vi "VOC_Multi-Sensor_Data_Logger.vi"() -> ()   [LabVIEW 2021]
uses:
  Program Files (x86)/National Instruments/LabVIEW 2021/examples/Instrument IO/Serial/support/Serial - XON-XOFF Characters.ctl
  Program Files (x86)/National Instruments/LabVIEW 2021/examples/Instrument IO/Serial/support/Serial - ASCII Characters.ctl
  Program Files (x86)/National Instruments/LabVIEW 2021/examples/Instrument IO/Serial/support/Serial - Settings.ctl
  <vilib>/Instr/_visa.llb/VISA Configure Serial Port (Instr).vi
  <vilib>/Utility/file.llb/Write Delimited Spreadsheet (string).vi
  <vilib>/Utility/file.llb/Write Delimited Spreadsheet (DBL).vi
panel:
  out "Elapsed Time (s)":i32
  in  "Log File":path=path "C:/Users/dfdye/Documents/GitHub/VOC_sensor_testing/Data_Logs/Test.tbd"
  in  "Data Logging Interval (sec)":i32=5 min=1 max=3600 step=1
  out "SGP30 TVOC (ppb)":dbl
  out "Humidity (%)":dbl
  out "Pressure (hPa)":dbl
  out "Temperature (deg C)":dbl
  in  "stop":bool
  in  "Serial Port":refnum<visa-resource-name>="COM3"
  out "XY Graph":cluster{i32[], dbl[]}[](graph)
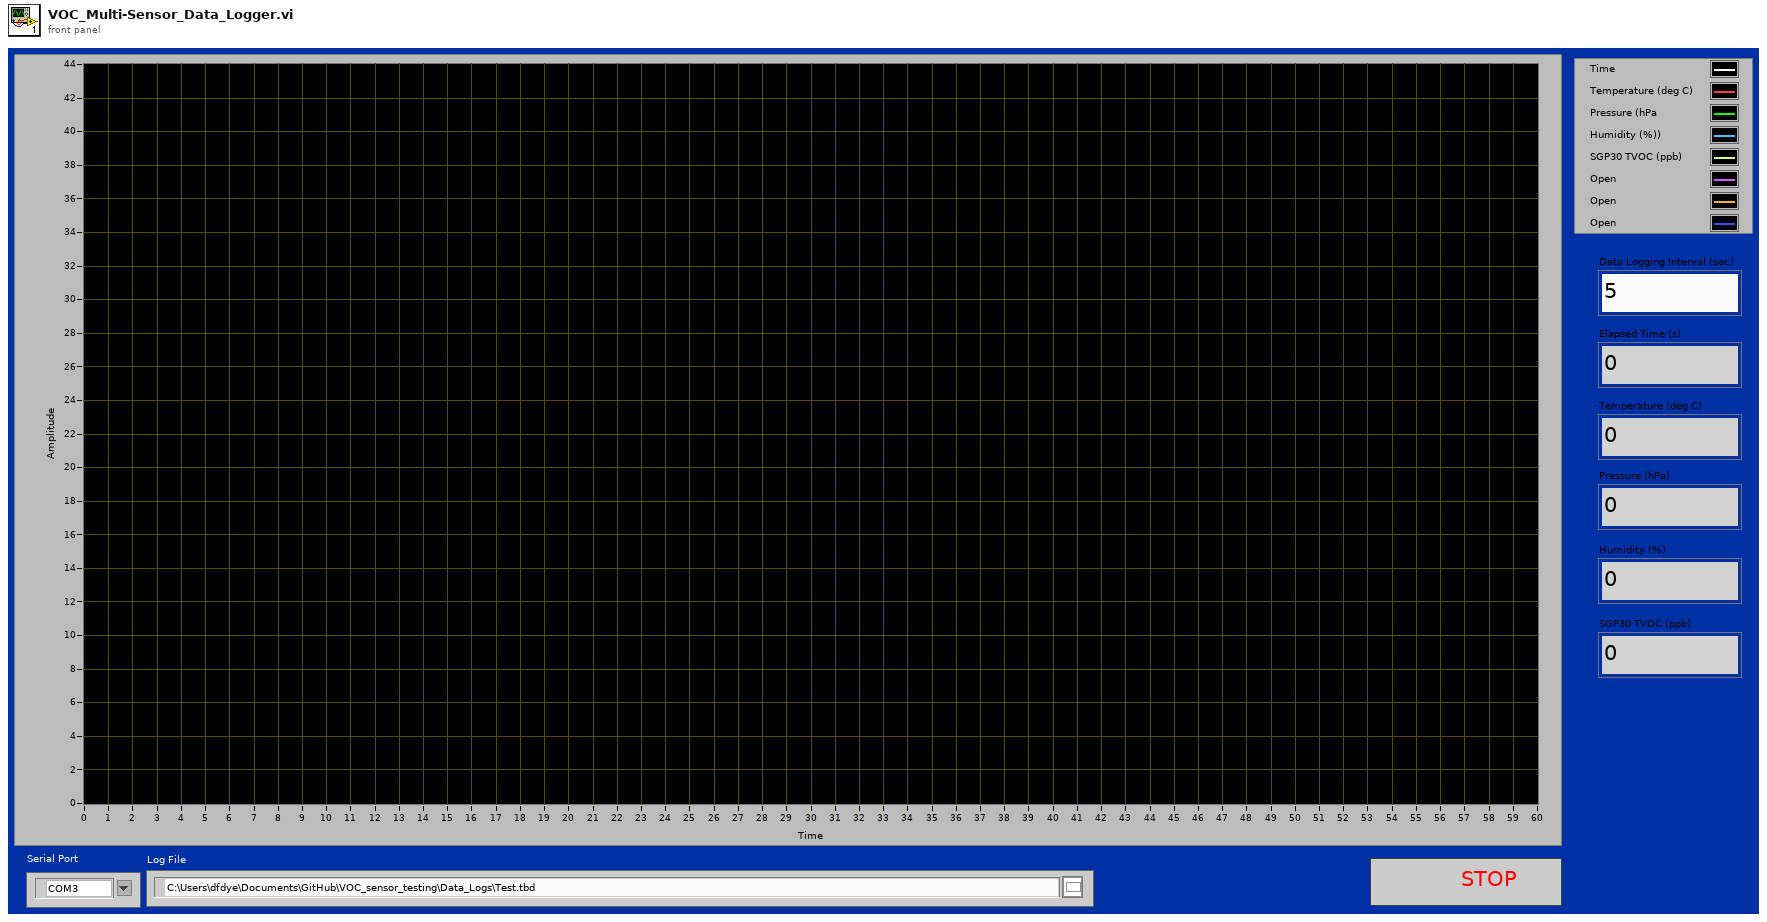
[diagram p1: front panel]
types:
  T1 = typedef "Serial - Settings.ctl" = cluster{"baud rate":u32, "data bits":u16, "parity":enum16{"None", "Odd", "Even", "Mark", "Space"}, "stop bits":u16, "flow control":u16}
  T2 = typedef "Serial - XON-XOFF Characters.ctl" = cluster{"XON":T3, "XOFF":T3}
  T3 = typedef "Serial - ASCII Characters.ctl" = enum16{"NUL", "SOH", "STX", "ETX", "EOT", "ENQ", "ACK", "BEL", "BS", "HT", "LF", "VT", "FF", "CR", "SO", "SI", "DLE", "DC1", "DC2", "DC3", "DC4", "NAK", "SYN", "ETB", "CAN", "EM", "SUB", "ESC", "FS", "GS", "RS", "US", "SP", "!", "\"", "#", "$", "%", "&", "'", "(", ")", "*", "+", ",", "- (-)", ".", "/", "0", "1", "2", "3", "4", "5", "6", "7", "8", "9", ":", ";", "<", "=", ">", "?", "@", "A", "B", "C", "D", "E", "F", "G", "H", "I", "J", "K", "L", "M", "N", "O", "P", "Q", "R", "S", "T", "U", "V", "W", "X", "Y", "Z", "[", "\\", "]", "^", "_", "`", "a", "b", "c", "d", "e", "f", "g", "h", "i", "j", "k", "l", "m", "n", "o", "p", "q", "r", "s", "t", "u", "v", "w", "x", "y", "z", "{", "|", "}", "~"}
  T4 = enum8{"Enabled", "Disabled", "Disabled and Grayed Out"}
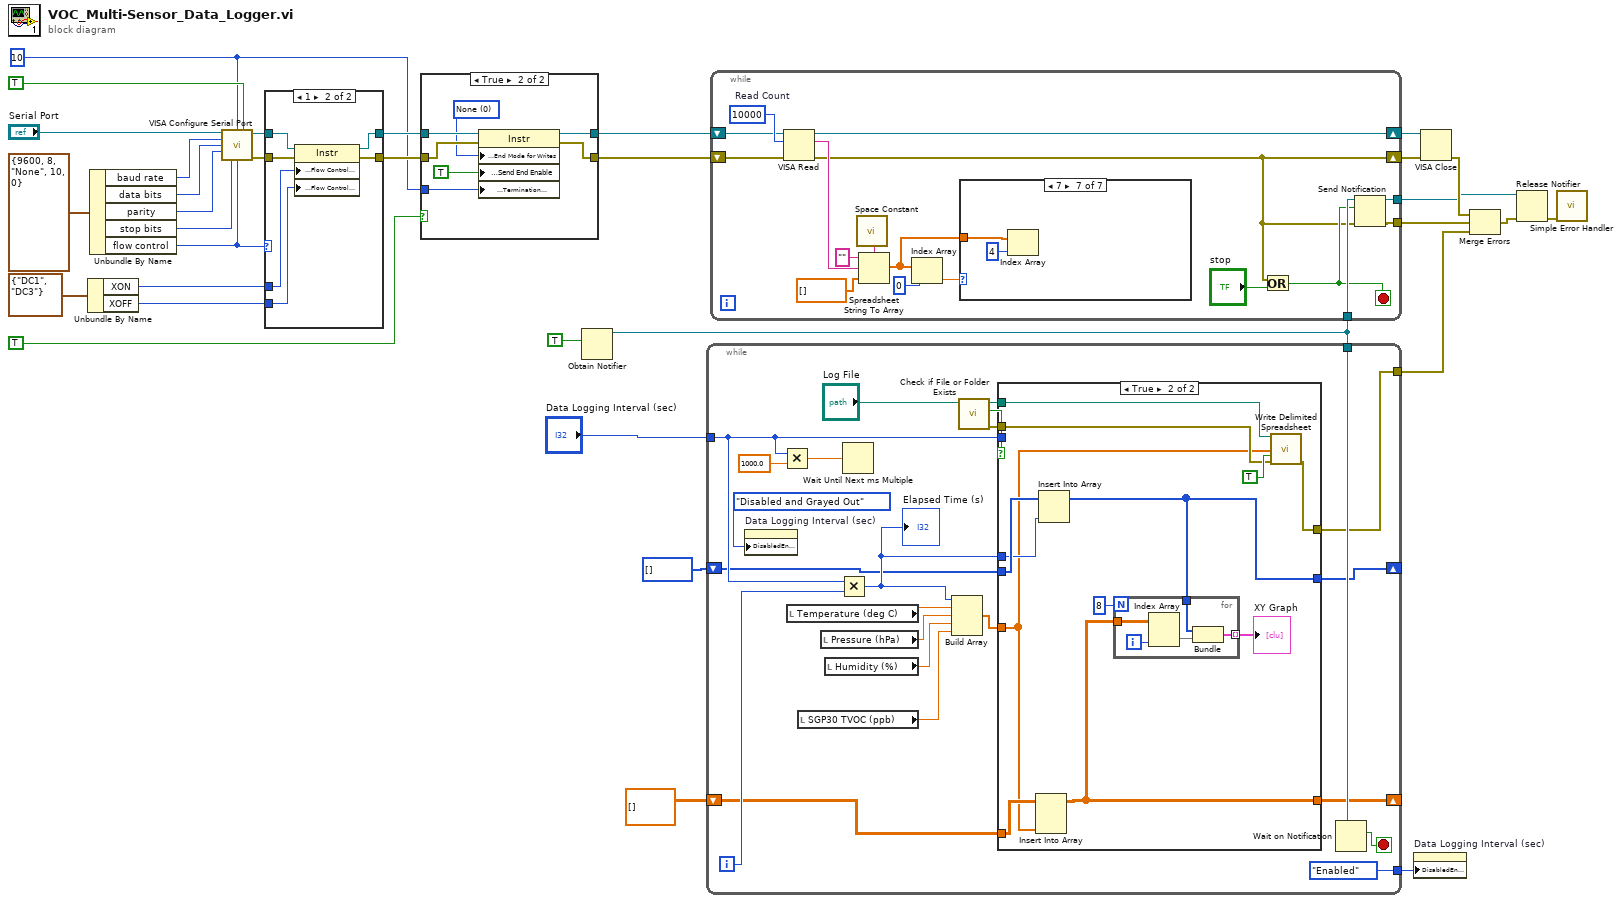
[diagram p0: block diagram]
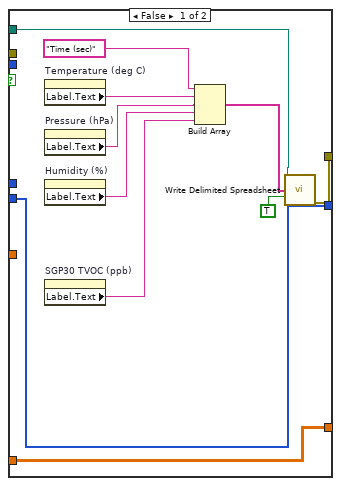
[diagram p2: hidden frame]
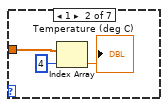
[diagram p4: hidden frame]
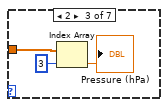
[diagram p5: hidden frame]
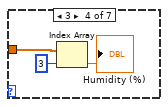
[diagram p6: hidden frame]
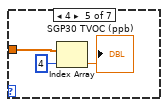
[diagram p7: hidden frame]
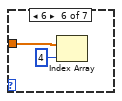
[diagram p8: hidden frame]
diagram:
  w17 = u8 10 ("Termination Character")
  n1 = Unbundle By Name(T2 {"XON"=enum."DC1", "XOFF"=enum."DC3"} ("XON/XOFF Characters")) -> ("XON"=w22:T3, "XOFF"=w21:T3)
  n2 = Unbundle By Name(T1 {"baud rate"=9600, "data bits"=8, "parity"=enum."None", "stop bits"=10, "flow control"=0} ("Serial Settings")) -> ("baud rate"=w26:u32, "data bits"=w27:u16, "parity"=w28:enum16{"None", "Odd", "Even", "Mark", "Space"}, "stop bits"=w29:u16, "flow control"=w23:u16)
  n3 = call-poly "VISA Configure Serial Port"("VISA resource name"="Serial Port", "termination char\n(0xA = '\\n' = LF)"=w17, "Enable Termination\nChar (T)"=TRUE ("End Read on Termination Character?"), "baud rate (9600)"=w26, "data bits (8)"=w27, "parity (0:none)"=w28, "stop bits (10: 1 bit)"=w29, "flow control (0:none)"=w23) -> ("VISA resource name out"=w30:refnum<visa-resource-name>, "error out"=w31:errorcluster)  [unwired: 2 in, 4 out]
  n4 = case shown="1" w23 {
    tunnel: [w34 w41] -> w20
    tunnel: [w35 w40] -> w19
    tunnel: w31 -> [w34 w39]
    tunnel: w30 -> [w35 w38]
    tunnel: w22 -> [_ w37]
    tunnel: w21 -> [_ w36]
    frame Default {
    }
    frame 1 {
      n5 = property class="Instr"(reference=w38, error in=w39, "Serial Settings:Flow Control XON Character"=w37, "Serial Settings:Flow Control XOFF Character"=w36) -> (reference out=w40:refnum<visa-resource-name>, error out=w41:errorcluster)
    }
  }
  n6 = case shown="True" TRUE ("End Write on Termination Character?") {
    tunnel: w19 -> [w42 w50]
    tunnel: w20 -> [w43 w49]
    tunnel: [w42 w48] -> w16
    tunnel: [w43 w47] -> w15
    tunnel: w17 -> [_ w45]
    frame False {
    }
    frame True {
      w46 = u16 0 items=["None", "LastBit", "TermChar", "Break"] ("Serial Settings:Serial End Mode for Writes")
      n7 = property class="Instr"(reference=w50, error in=w49, "Serial Settings:End Mode for Writes"=w46, "Message Based Settings:Send End Enable"=TRUE, "Message Based Settings:Termination Character"=w45) -> (reference out=w48:refnum<visa-resource-name>, error out=w47:errorcluster)
    }
  }
  n8 = Obtain Notifier(notification data type=TRUE) -> (notifier out=w6:refnum<notifier>)  [unwired: 3 in, 2 out]
  n9 = while {
    tunnel: w6 -> [w72]
    tunnel: [w61] -> w5
    tunnel: "Data Logging Interval (sec)" -> [w57]
    tunnel: [T4."Enabled" ("Disabled")] -> w3
    shift-right: [w55] -> _
    shift-left: dbl[][] [] -> [w56]
    shift-right: [w53] -> _
    shift-left: i32[] [] -> [w52]
    i -> [w58]
    stop <- w73 stop-if-true
    n10 = property on="Data Logging Interval (sec)" class="DigNum (strict)"("DisabledEnum"=T4."Disabled and Grayed Out" ("Disabled")) -> ()  [unwired: 2 in, 2 out]
    n11 = Multiply(x=w57, y=1000.0) -> (x*y=w71:dbl)
    n12 = local read "Temperature (deg C)"() -> (w67:dbl)
    n13 = local read "SGP30 TVOC (ppb)"() -> (w51:dbl)
    n14 = local read "Pressure (hPa)"() -> (w68:dbl)
    n15 = local read "Humidity (%)"() -> (w69:dbl)
    n16 = Multiply(x=w57, y=w58) -> (x*y=w54:i32)
    "Elapsed Time (s)" <- w54
    n17 = Wait Until Next ms Multiple(millisecond multiple=w71) -> ()  [unwired: 1 out]
    n18 = Build Array(w54, w67, w68, w69, w51) -> (w66:dbl[])
    n19 = call <vilib>:"Check if File or Folder Exists.vi"("path"="Log File") -> ("error out"=w62:errorcluster, "file or folder exists?"=w63:bool, "dup path"=w64:path)  [unwired: 8 in]
    n20 = case shown="True" w63 {
      tunnel: w66 -> [_ w85]
      tunnel: w64 -> [w78 w95]
      tunnel: w62 -> [_ w94]
      tunnel: [w83 w93] -> w61
      tunnel: w57 -> [_ _]
      tunnel: w56 -> [w76 w92]
      tunnel: [w76 w87] -> w55
      tunnel: [w75 w86] -> w53
      tunnel: w54 -> [_ w90]
      tunnel: w52 -> [w75 w91]
      frame False {
        n21 = property on="Temperature (deg C)" class="DigNum (strict)"() -> ("Label.Text"=w82:string)  [unwired: 2 in, 2 out]
        n22 = property on="Pressure (hPa)" class="DigNum (strict)"() -> ("Label.Text"=w81:string)  [unwired: 2 in, 2 out]
        n23 = property on="Humidity (%)" class="DigNum (strict)"() -> ("Label.Text"=w80:string)  [unwired: 2 in, 2 out]
        n24 = property on="SGP30 TVOC (ppb)" class="DigNum (strict)"() -> ("Label.Text"=w74:string)  [unwired: 2 in, 2 out]
        n25 = Build Array("Time (sec)" ("element"), w82, w81, w80, w74) -> (w79:string[])
        n26 = call-poly <vilib>:"Write Delimited Spreadsheet.vi"("file path (dialog if empty)"=w78, "1D data"=w79, "append to file? (new file:F)"=TRUE) -> ("error out"=w83:errorcluster)  [unwired: 11 in, 1 out]
      }
      frame True {
        n27 = Insert Into Array(array=w92, new element=w85) -> (w87:dbl[][])  [unwired: 2 in]
        n28 = Insert Into Array(array=w91, new element=w90) -> (w86:i32[])  [unwired: 1 in]
        n29 = for {
          N: 8 -> [_]
          tunnel: [w99] -> w88 mode=indexing
          tunnel: w87 -> [w98]
          tunnel: w86 -> [w97]
          i -> [w101]
          n30 = Index Array(array=w98, index (col)=w101) -> (element=w100:dbl[])  [unwired: 1 in]
          n31 = Bundle(w97, w100) -> (w99:cluster{i32[], dbl[]})  [unwired: 1 in]
        }
        "XY Graph" <- w88
        n32 = call-poly <vilib>:"Write Delimited Spreadsheet.vi"("file path (dialog if empty)"=w95, "1D data"=w85, "append to file? (new file:F)"=TRUE, "error in (no error)"=w94) -> ("error out"=w93:errorcluster)  [unwired: 10 in, 1 out]
      }
    }
    n33 = Wait on Notification(notifier=w72) -> (notification=w73:bool)  [unwired: 3 in, 3 out]
  }
  n34 = while {
    shift-right: [w115] -> w14
    shift-left: w16 -> [w117]
    shift-right: [w104] -> w13
    shift-left: w15 -> [w116]
    tunnel: w6 -> [w106]
    tunnel: [w103] -> w11
    tunnel: [w102] -> w7
    stop <- w105 stop-if-true
    w118 = u32 10000  # Read Count
    n35 = VISA Read(VISA resource name=w117, byte count=w118, error in (no error)=w116) -> (VISA resource name out=w115:refnum<visa-resource-name>, read buffer=w108:string, error out=w104:errorcluster)  [unwired: 1 out]
    n36 = call <vilib>:"Space Constant.vi"() -> ("String"=w114:string)
    n37 = Spreadsheet String To Array(delimiter (Tab)=w114, format string="", spreadsheet string=w108, array type (2D Dbl)=dbl[] []) -> (array=w109:dbl[])
    n38 = Index Array(array=w109, index=0) -> (element=w110:dbl)
    n39 = case shown="7" w110 {
      tunnel: w109 -> [_ w121 w124 w127 w130 w132 w134]
      frame 0, Default {
      }
      frame 1 {
        n40 = Index Array(array=w121, index=4) -> (element=→"Temperature (deg C)":dbl)
      }
      frame 2 {
        n41 = Index Array(array=w124, index=3) -> (element=→"Pressure (hPa)":dbl)
      }
      frame 3 {
        n42 = Index Array(array=w127, index=3) -> (element=→"Humidity (%)":dbl)
      }
      frame 4 {
        n43 = Index Array(array=w130, index=4) -> (element=→"SGP30 TVOC (ppb)":dbl)
      }
      frame 6 {
        n44 = Index Array(array=w132, index=4) -> ()  [unwired: 1 out]
      }
      frame 7 {
        n45 = Index Array(array=w134, index=4) -> ()  [unwired: 1 out]
      }
    }
    n46 = Or(x=w104, y="stop") -> (x .or. y?=w105:bool)
    n47 = Send Notification(notification=w105, notifier=w106, error in (no error)=w104) -> (notifier out=w102:refnum<notifier>, error out=w103:errorcluster)
  }
  n48 = property on="Data Logging Interval (sec)" class="DigNum (strict)"("DisabledEnum"=w3) -> ()  [unwired: 2 in, 2 out]
  n49 = VISA Close(VISA resource name=w14, error in (no error)=w13) -> (error out=w10:errorcluster)
  n50 = Merge Errors(w10, w11, w5) -> (w8:errorcluster)
  n51 = Release Notifier(notifier=w7, error in (no error)=w8) -> (error out=w9:errorcluster)  [unwired: 1 in, 2 out]
  n52 = call <vilib>:"Simple Error Handler.vi"("error in (no error)"=w9) -> ()  [unwired: 1 in, 8 out]
